vi "Teleop.vi"(10 "Match Info":T1={"Autonomous Elapsed Seconds"=0.0, "TeleOp Elapsed Seconds"=0.0, "Disabled Elapsed Seconds"=0.0, "Visited Autonomous"=FALSE, "Visited TeleOp"=FALSE, "Visited Disabled"=FALSE, "Autonomous Settings"={"Autonomous Style"=enum."Independent", "VI Refnum"=refnum}}, 11 "Call Context":T2) -> ()   [LabVIEW 2019]
doc: "This VI is called for each enabled TeleOp packet received from the DS. It is typically used to read from joysticks and other inputs and update I/O or setpoints for timed control loops. It should complete and return within 20 milliseconds or risk missing DS packets."
uses:
  <vilib>/Rock Robotics/WPI/DriverStation/WPI_DriverStationDerivedRobotMode.ctl
  <vilib>/Rock Robotics/WPI/DriverStation/WPI_DriverStationMatch Info.ctl
  <vilib>/Rock Robotics/WPI/DriverStation/WPI_DriverStationRobotMode2.ctl
  <vilib>/Rock Robotics/WPI/Utilities/WPI_GetSetVariantRefNum.vi
  <vilib>/Rock Robotics/Network Tables/NT Read Number.vi
  Framework/Robot Global Data.vi
  <vilib>/Rock Robotics/Network Tables/NT Write Number.vi
panel:
  out "Ta":dbl
  out "Tx":dbl
  in  "Limelight ON?":bool
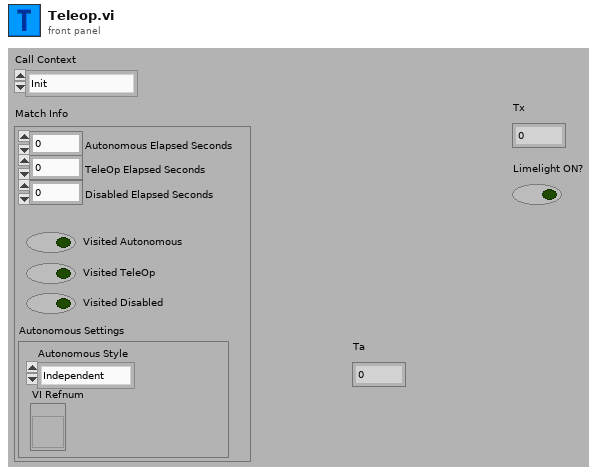
[diagram p1: front panel]
types:
  T1 = typedef "WPI_DriverStationMatch Info.ctl" = cluster{"Autonomous Elapsed Seconds":dbl, "TeleOp Elapsed Seconds":dbl, "Disabled Elapsed Seconds":dbl, "Visited Autonomous":bool, "Visited TeleOp":bool, "Visited Disabled":bool, "Autonomous Settings":cluster{"Autonomous Style":enum16{"Iterative", "Independent"}, "VI Refnum":refnum<vi>}}
  T2 = typedef "WPI_DriverStationDerivedRobotMode.ctl" = enum16{"Init", "Execute", "Stop"}
  T3 = typedef "WPI_DriverStationRobotMode2.ctl" = enum16{"Autonomous Disabled", "Autonomous Enabled", "Teleop Disabled", "Teleop Enabled", "Disconnected", "Finish", "Test Disabled", "Test Enabled", "Emergency Stopped"}
  T4 = typedef "WPI_JoystickDevRef.ctl" = cluster{"Device":T5}
  T5 = typedef "WPI_JoystickDeviceEnum.ctl" = enum16{"USB 0", "USB 1", "USB 2", "USB 3", "USB 4", "USB 5"}
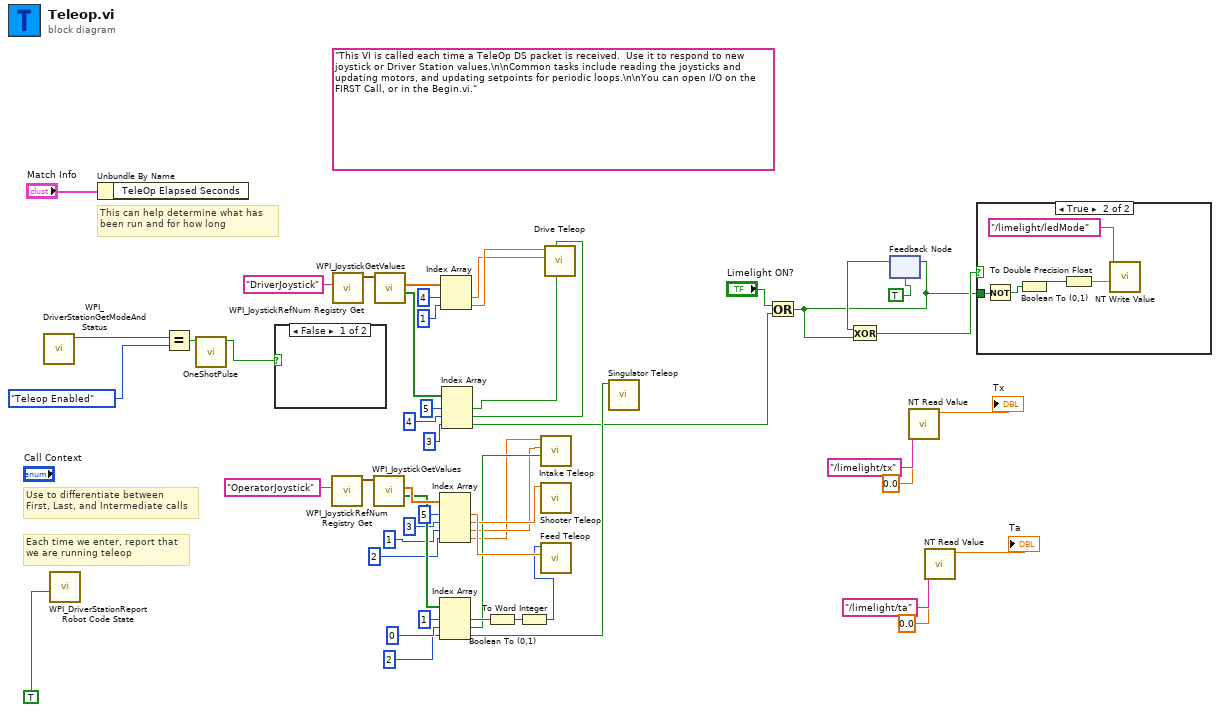
[diagram p0: block diagram]
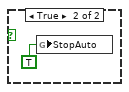
[diagram p2: hidden frame]
diagram:
  (unwired) "This VI is called each time a TeleOp DS packet is received.  Use it to respond to new joystick or Driver Station values.\n\nCommon tasks include reading the joysticks and updating motors, and updating setpoints for periodic loops.\n\nYou can open I/O on the FIRST Call, or in the Begin.vi."
  # "Each time we enter, report that\nwe are running teleop"
  # "Use to differentiate between\nFirst, Last, and Intermediate calls"
  # "This can help determine what has\nbeen run and for how long"
  n1 = call <vilib>:"WPI_DriverStationGetModeAndStatus.vi"() -> ("Robot Mode"=w4:T3)  [unwired: 10 in, 1 out]
  n2 = call <vilib>:"WPI_DriverStationReport Robot Code State.vi"("TeleOp"=TRUE ("Autonomous")) -> ()  [unwired: 10 in, 1 out]
  n3 = Unbundle By Name("Match Info") -> ()  [unwired: 1 out]
  n4 = Equal?(x=w4, y=WPI_DriverStationRobotMode2."Teleop Enabled" ("Robot Mode")) -> (x = y?=w2:bool)
  n5 = call "OneShotPulse.vi"("Input"=w2) -> ("Output"=w1:bool)  [unwired: 10 in]
  n6 = case shown="False" w1 {
    frame False {
    }
    frame True {
      n7 = global write "Robot Global Data.vi" "StopAuto"(TRUE) -> ()
    }
  }
  n8 = call <vilib>:"WPI_JoystickRefNum Registry Get.vi"("refnum name"="OperatorJoystick") -> ("JoystickDevRef"=w41:T4)  [unwired: 9 in, 1 out]
  n9 = call <vilib>:"WPI_JoystickRefNum Registry Get.vi"("refnum name"="DriverJoystick") -> ("JoystickDevRef"=w49:T4)  [unwired: 9 in, 1 out]
  n10 = call <vilib>:"WPI_JoystickGetValues.vi"("JoystickDevRef"=w41) -> ("Buttons"=w34:bool[], "Axes"=w35:dbl[])  [unwired: 6 in, 3 out]
  n11 = call <vilib>:"WPI_JoystickGetValues.vi"("JoystickDevRef"=w49) -> ("Buttons"=w45:bool[], "Axes"=w48:dbl[])  [unwired: 6 in, 3 out]
  n12 = Index Array(array=w35, index #1=5 ("index"), index #2=3 ("index"), index #3=1, index #4=2) -> (element #1=w31:dbl, element #2=w26:dbl, element #3=w21:dbl, element #4=w20:dbl)
  n13 = Index Array(array=w34, index #1=1 ("index"), index #2=0, index #3=2) -> (element #1=w30:bool, element #2=w24:bool, element #3=w18:bool)
  n14 = Index Array(array=w48, index #1=4 ("index"), index #2=1 ("index")) -> (element #1=w39:dbl, element #2=w40:dbl)
  n15 = Index Array(array=w45, index #1=5 ("index"), index #2=4 ("index"), index #3=3 ("index")) -> (element #1=w38:bool, element #2=w37:bool, element #3=w12:bool)
  n16 = Boolean To (0,1)(Boolean=w30) -> (0, 1=w29:i16)
  n17 = To Word Integer(number=w29) -> (16bit integer=w28:i16)
  n18 = call "Intake Teleop.vi"("Toggle Flip"=w24, "Intake Lift"=w21, "Wheel Speed"=w20) -> ()  [unwired: 9 in]
  n19 = call "Shooter Teleop.vi"("Setpoint"=w26) -> ()  [unwired: 11 in]
  n20 = call "Feed Teleop.vi"("Elevator"=w31, "Feed Wheel"=w28) -> ()  [unwired: 10 in]
  n21 = call "Drive Teleop.vi"("Quick Turn"=w38, "Auto Align"=w37, "Wheel"=w39, "Throttle"=w40) -> ()  [unwired: 8 in]
  n22 = call "Singulator Teleop.vi"("Setpoint"=w18) -> ()  [unwired: 11 in]
  n23 = Or(x="Limelight ON?", y=w12) -> (x .or. y?=w11:bool)
  n24 = feedback-in #1(w11) -> ()
  n25 = feedback #1(TRUE) -> (w16:bool)
  n26 = Exclusive Or(1:w11, 2:w16) -> (0:w15:bool)
  n27 = call-poly <vilib>:"NT Read Value.vi"("Default Value"=0.0, "Name"="/limelight/tx") -> ("Numeric"=→"Tx":dbl)  [unwired: 8 in, 1 out]
  n28 = call-poly <vilib>:"NT Read Value.vi"("Default Value"=0.0, "Name"="/limelight/ta") -> ("Numeric"=→"Ta":dbl)  [unwired: 8 in, 1 out]
  n29 = case shown="True" w15 {
    tunnel: w11 -> [_ w54]
    frame False {
    }
    frame True {
      n30 = Not(x=w54) -> (.not. x?=w53:bool)
      n31 = Boolean To (0,1)(Boolean=w53) -> (0, 1=w56:i16)
      n32 = To Double Precision Float(number=w56) -> (double precision float=w55:dbl)
      n33 = call-poly <vilib>:"NT Write Value.vi"("Numeric"=w55, "Name"="/limelight/ledMode") -> ()  [unwired: 9 in, 1 out]
    }
  }
